vi "Open VI.vi"(0 "Logic VI Path":path, 11 "error in (no error)":errorcluster) -> (15 "error out":errorcluster)   [LabVIEW 2021, in "Converter.lvlib"]
uses:
  Converter.lvlib
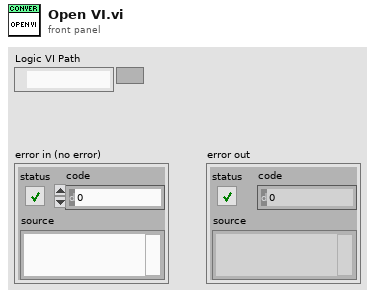
[diagram p1: front panel]
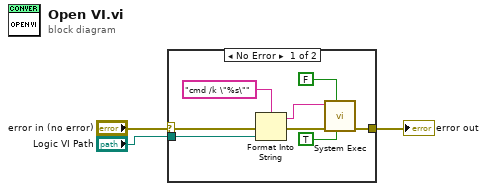
[diagram p0: block diagram]
diagram:
  n1 = case shown="No Error" "error in (no error)" {
    selector: "error in (no error)" -> [w5 w12]
    tunnel: [w11 w12] -> w3
    tunnel: "Logic VI Path" -> [w4 _]
    frame No Error {
      n2 = Format Into String(format string="cmd /k \"%s\"", error in=w5, w4) -> (resulting string=w7:string, error out=w10:errorcluster)  [unwired: 1 in]
      n3 = call <vilib>:"System Exec.vi"("run minimized? (F)"=TRUE, "wait until completion? (T)"=FALSE, "error in (no error)"=w10, "command line"=w7) -> ("error out"=w11:errorcluster)  [unwired: 4 in, 3 out]
    }
    frame Error {
    }
  }
  "error out" <- w3
